vi "Day 25.vi"() -> ()   [LabVIEW 2023]
panel:
  out "Array size":i32
  out "SNAFU sum":string
  out "decimal to SNAFU":string[](array[string])
  out "sum":dbl format="%#_6f"
  out "Decimal array":dbl[](array[numeric]) format="%#_6f"
  out "SNAFU  array":string[](array[string])
  in  "String":string="1--20\n1-00==1-1==\n12011==21020=-2021-\n101--=11\n22-=02=\n112=12-222\n10=-0-=10\n202-1-20=01-10-2\n11==\n122==1=100-\n1====2==121--=1\n1=-02-=011-2=2-00=00\n1000=2\n12-\n201=2-1-1=02--=1=1\n1=01-1=-1=012-2-=\n1=1=\n11102\n10=\n2-=--2=2=-==11-11\n2=02\n10-1-00=0-20\n1-0=11=\n2=1=0=1022=-\n1==1--2-=02=\n1=12-2\n200-\n20=02-211=11=\n1==12=-0-\n1=1-0101=-1\n2=21000-22\n1--1=11-2-=1--211-\n2-=101=-\n1-20210-0-1=101=1\n1===1===-\n211=2-0==\n21===1==0\n10\n2=0-1=110221-2-2\n1001220120=-=\n10=21=0-=--=21-=\n1=0=1-2-0\n21-0===21=2100-02\n1=-=0-0-12=-0--202=\n101200-111--10-=-\n2201==0--=-\n12-02201-====-=\n2-1220-\n10-\n2=00-2-2\n22-\n1=01--==\n202-11..."
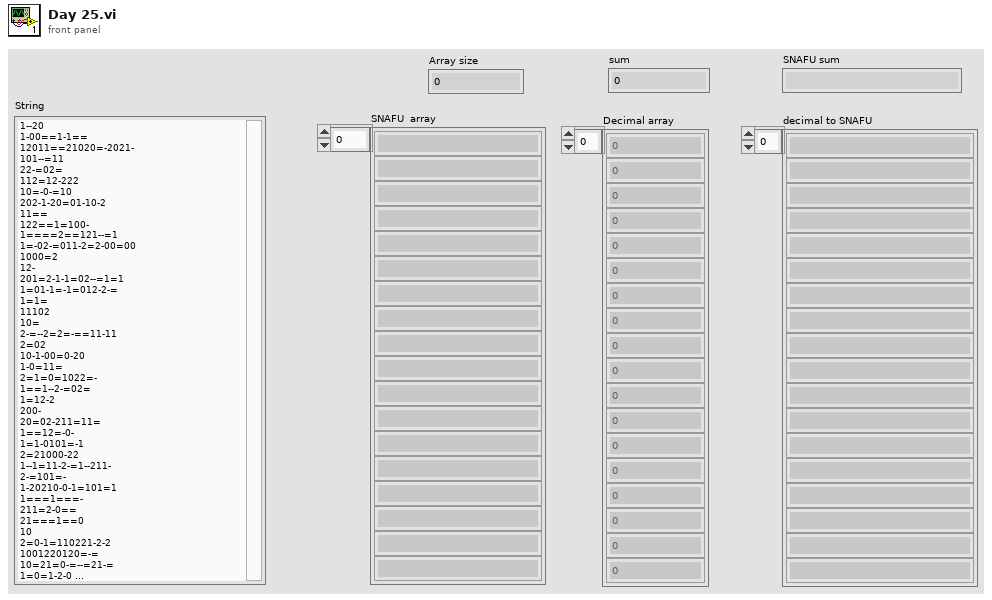
[diagram p1: front panel]
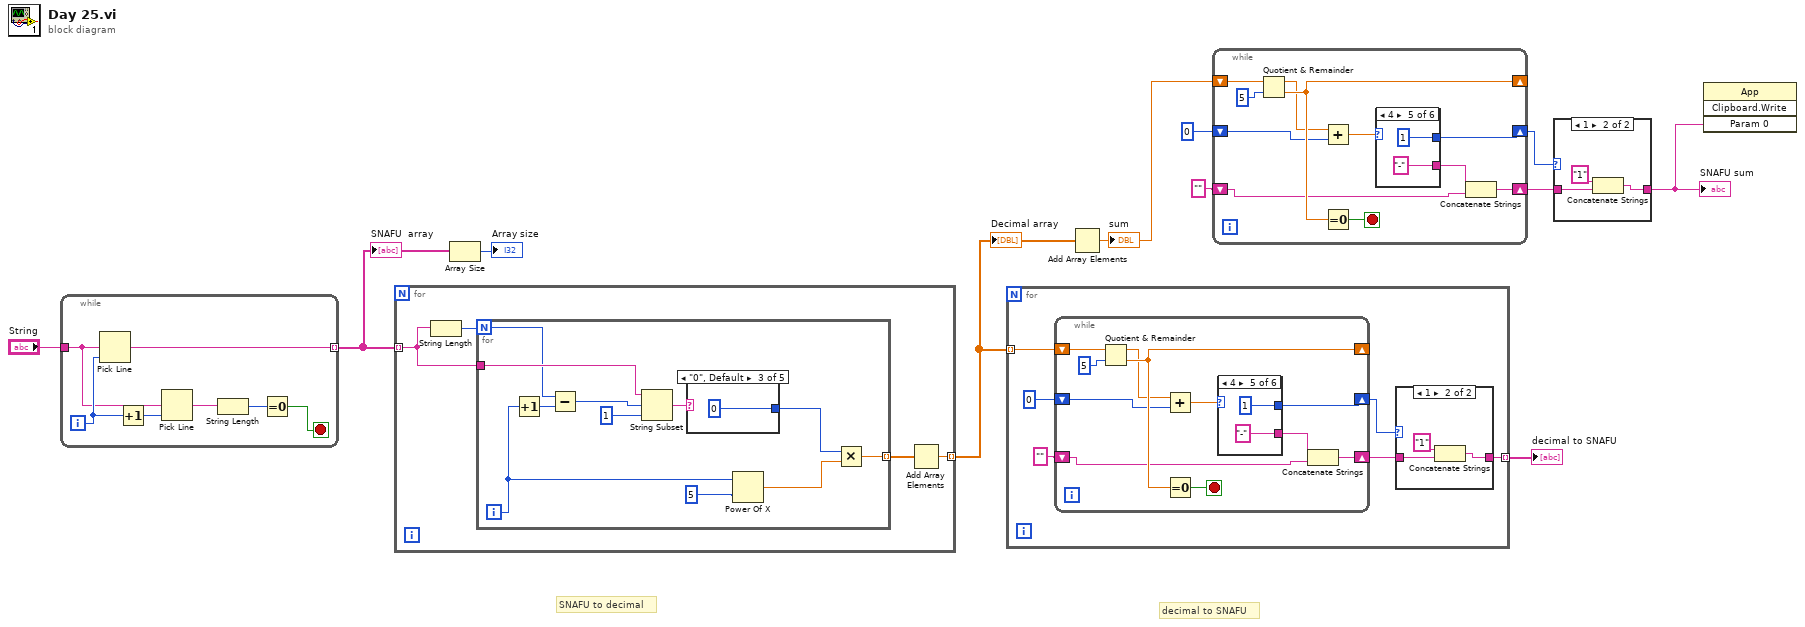
[diagram p0: block diagram]
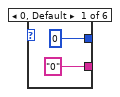
[diagram p3: hidden frame]
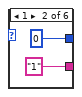
[diagram p4: hidden frame]
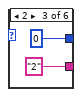
[diagram p5: hidden frame]
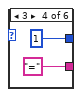
[diagram p6: hidden frame]
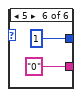
[diagram p7: hidden frame]
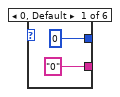
[diagram p9: hidden frame]
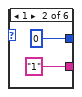
[diagram p10: hidden frame]
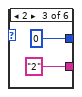
[diagram p11: hidden frame]
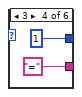
[diagram p12: hidden frame]
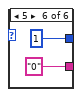
[diagram p13: hidden frame]
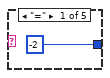
[diagram p14: hidden frame]
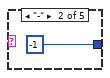
[diagram p15: hidden frame]
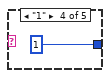
[diagram p16: hidden frame]
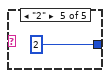
[diagram p17: hidden frame]
diagram:
  # "decimal to SNAFU"
  # "SNAFU to decimal"
  n1 = while {
    tunnel: "String" -> [w14]
    tunnel: [w17] -> w4 mode=indexing
    i -> [w15]
    stop <- w12 stop-if-true
    n2 = Pick Line(multi-line string=w14, line index=w15) -> (output string=w17:string)  [unwired: 1 in]
    n3 = Increment(x=w15) -> (x+1=w13:i32)
    n4 = Pick Line(multi-line string=w14, line index=w13) -> (output string=w16:string)  [unwired: 1 in]
    n5 = String Length(string=w16) -> (length=w18:i32)
    n6 = Equal To 0?(x=w18) -> (x = 0?=w12:bool)
  }
  "SNAFU  array" <- w4
  n7 = for {
    tunnel: w4 -> [w21] mode=indexing
    tunnel: [w19] -> w10 mode=indexing
    n8 = String Length(string=w21) -> (length=w22:i32)
    n9 = for {
      N: w22 -> [w27]
      tunnel: w21 -> [w32]
      tunnel: [w28] -> w20 mode=indexing
      i -> [w26]
      n10 = Increment(x=w26) -> (x+1=w25:i32)
      n11 = Subtract(x=w27, y=w25) -> (x-y=w24:i32)
      n12 = String Subset(string=w32, offset (0)=w24, length (rest)=1 ("length (rest)")) -> (substring=w31:string)
      n13 = case shown="\"0\", Default" w31 {
        tunnel: [-2 ("length (rest)") -1 ("length (rest)") i64 0 ("length (rest)") 1 ("length (rest)") 2 ("length (rest)")] -> w29
        frame "=" {
        }
        frame "-" {
        }
        frame "0", Default {
        }
        frame "1" {
        }
        frame "2" {
        }
      }
      n14 = Power Of X(1:5 ("x"), 2:w26) -> (0:w23:dbl)
      n15 = Multiply(x=w29, y=w23) -> (x*y=w28:dbl)
    }
    n16 = Add Array Elements(numeric array=w20) -> (sum=w19:dbl)
  }
  "Decimal array" <- w10
  n17 = Array Size(array=w4) -> (size(s)=→"Array size":i32)
  n18 = for {
    tunnel: w10 -> [w44] mode=indexing
    tunnel: [w39] -> w1 mode=indexing
    n19 = while {
      shift-right: [w56] -> _
      shift-left: w44 -> [w58]
      shift-right: [w50] -> w41
      shift-left: "" -> [w49]
      shift-right: [w54] -> w40
      shift-left: 0 ("Numeric") -> [w52]
      stop <- w57 stop-if-true
      n20 = Quotient & Remainder(x=w58, y=5) -> (x-y*floor(x/y)=w55:dbl, floor(x/y)=w56:dbl)
      n21 = Add(x=w55, y=w52) -> (x+y=w53:dbl)
      n22 = Equal To 0?(x=w56) -> (x = 0?=w57:bool)
      n23 = case shown="4" w53 {
        tunnel: [0 ("Numeric") 0 ("Numeric") 0 ("Numeric") 1 ("Numeric") 1 ("Numeric") 1 ("Numeric")] -> w54
        tunnel: ["0" "1" "2" "=" "-" "0"] -> w51
        frame 0, Default {
        }
        frame 1 {
        }
        frame 2 {
        }
        frame 3 {
        }
        frame 4 {
        }
        frame 5 {
        }
      }
      n24 = Concatenate Strings(w51, w49) -> (w50:string)
    }
    n25 = case shown="1" w40 {
      tunnel: w41 -> [w45 w48]
      tunnel: [w45 w47] -> w39
      frame 0, Default {
      }
      frame 1 {
        n26 = Concatenate Strings("1" ("string"), w48) -> (w47:string)
      }
    }
  }
  "decimal to SNAFU" <- w1
  n27 = Add Array Elements(numeric array=w10) -> (sum=w5:dbl)
  "sum" <- w5
  n28 = while {
    shift-right: [w79] -> _
    shift-left: w5 -> [w81]
    shift-right: [w73] -> w8
    shift-left: "" -> [w72]
    shift-right: [w77] -> w9
    shift-left: 0 ("Numeric") -> [w75]
    stop <- w80 stop-if-true
    n29 = Quotient & Remainder(x=w81, y=5) -> (x-y*floor(x/y)=w78:dbl, floor(x/y)=w79:dbl)
    n30 = Add(x=w78, y=w75) -> (x+y=w76:dbl)
    n31 = Equal To 0?(x=w79) -> (x = 0?=w80:bool)
    n32 = case shown="4" w76 {
      tunnel: [0 ("Numeric") 0 ("Numeric") 0 ("Numeric") 1 ("Numeric") 1 ("Numeric") 1 ("Numeric")] -> w77
      tunnel: ["0" "1" "2" "=" "-" "0"] -> w74
      frame 0, Default {
      }
      frame 1 {
      }
      frame 2 {
      }
      frame 3 {
      }
      frame 4 {
      }
      frame 5 {
      }
    }
    n33 = Concatenate Strings(w74, w72) -> (w73:string)
  }
  n34 = case shown="1" w9 {
    tunnel: w8 -> [w95 w98]
    tunnel: [w95 w97] -> w2
    frame 0, Default {
    }
    frame 1 {
      n35 = Concatenate Strings("1" ("string"), w98) -> (w97:string)
    }
  }
  "SNAFU sum" <- w2
  n36 = invoke class="App" method="Clipboard.Write"("Param 0"=w2) -> ()  [unwired: 3 in, 4 out]
